vi "Define Ref Curve Panel.vi"(8 "error in (no error)":errorcluster caption="错误输入（无错误）", 10 "parentPanelHandle":i32, 11 "asicHandle":i32) -> (0 "error out":errorcluster caption="错误输出", 3 "function return":i32)   [LabVIEW 2018]
doc: "extern int __stdcall APSxDefineRefCurvePanel (int asicHandle, IN int parentPanelHandle);"
uses:
  APSx.dll/APSx.dll
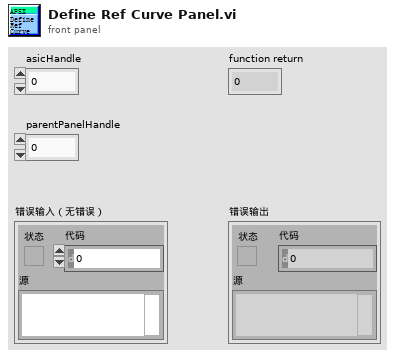
[diagram p1: front panel]
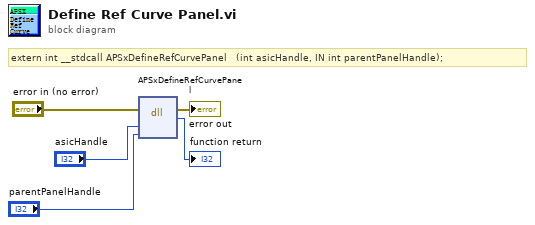
[diagram p0: block diagram]
diagram:
  # "extern int __stdcall APSxDefineRefCurvePanel   (int asicHandle, IN int parentPanelHandle);"
  n1 = dll-call lib="PTH2[abs D项目Feng恒隆项目Labview传感器对中台SourcesAPSx.dllAPSx.*" fn="APSxDefineRefCurvePanel"(error in="error in (no error)", "asicHandle"="asicHandle", "parentPanelHandle"="parentPanelHandle") -> (error out=→"error out":errorcluster, →"function return":i32)  [unwired: 4 in, 1 out]
